vi "Add Column.vi"(8 "error in (no error)":errorcluster, 9 "Data[]":string[](array[string]), 10 "Header":string, 11 "SLL Table in":refnum<class "SLL Table.lvclass">) -> (0 "error out":errorcluster, 3 "SLL Table out":refnum<class "SLL Table.lvclass">)   [LabVIEW 2016, in "SLL Table.lvclass"]
doc: "Add a new column by specifying the header and the data for it."
uses:
  SLL Table.lvclass
  SLL Table.lvclass/SLL Table.ctl
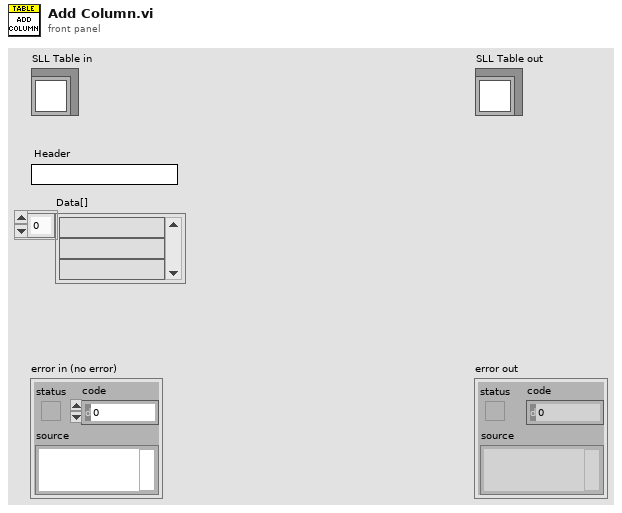
[diagram p1: front panel]
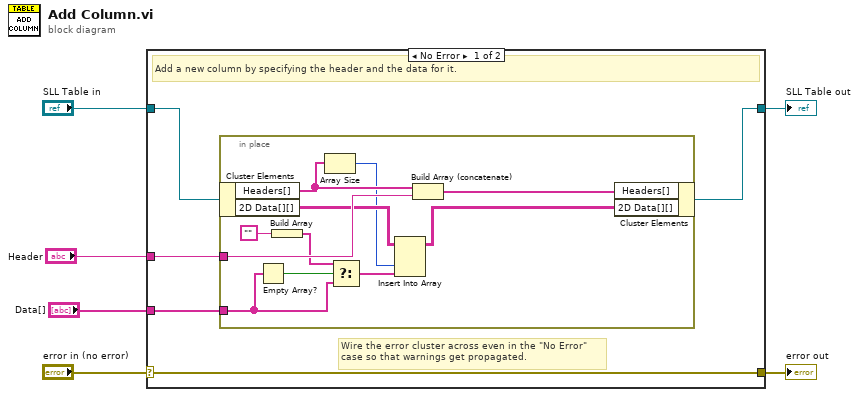
[diagram p0: block diagram]
diagram:
  n1 = case shown="No Error" "error in (no error)" {
    selector: "error in (no error)" -> [w11 w24]
    tunnel: [w11 w24] -> w5
    tunnel: [w7 w23] -> w3
    tunnel: "SLL Table in" -> [w10 w23]
    tunnel: "Header" -> [w9 _]
    tunnel: "Data[]" -> [w8 _]
    frame No Error {
      # "Wire the error cluster across even in the \"No Error\"\ncase so that warnings get propagated."
      # "Add a new column by specifying the header and the data for it."
      n2 = in-place "In Place Element Structure" {
        in-place-border: w9 -> [w22]
        in-place-border: w8 -> [w19]
        n3 = in-place-cluster #1(w10) -> ("Headers[]"=w13:string[], "2D Data[][]"=w16:string[][])
        n4 = Empty Array?(array=w19) -> (empty?=w20:bool)
        n5 = Build Array("" ("Empty String Constant")) -> (w17:string[])
        n6 = Array Size(array=w13) -> (size(s)=w12:i32)
        n7 = Select(t=w17, s=w20, f=w19) -> (s? t:f=w15:string[])
        n8 = Insert Into Array(array=w16, index (col)=w12, new element=w15) -> (w14:string[][])  [unwired: 1 in]
        n9 = Build Array (concatenate)(w13, w22) -> (w21:string[])
        n10 = in-place-cluster #1("Headers[]"=w21, "2D Data[][]"=w14) -> (w7:refnum<class "SLL Table.lvclass">)
      }
    }
    frame Error {
    }
  }
  "error out" <- w5
  "SLL Table out" <- w3
